vi "LVClass_HasoSlopes ctor from HasoData.vi"(0 "HasoSlopes (new)":refnum<class "HasoSlopes.lvclass">, 5 "HasoData":refnum<class "HasoData.lvclass">, 7 "Slopes?":enum16{"raw_slopes", "processed_slopes"}(ring), 11 "error in (no error)":errorcluster) -> (4 "HasoSlopes (new)":refnum<class "HasoSlopes.lvclass">, 6 "HasoData (dup)":refnum<class "HasoData.lvclass">, 15 "error out":errorcluster)   [LabVIEW 2020, in "HasoSlopes.lvclass"]
uses:
  HasoSlopes.lvclass
  HasoData.lvclass
  Handle creation.ctl
  HasoSlopes.lvclass/HasoSlopes.ctl
  LVClass_HasoData Read HasoData - property.vi
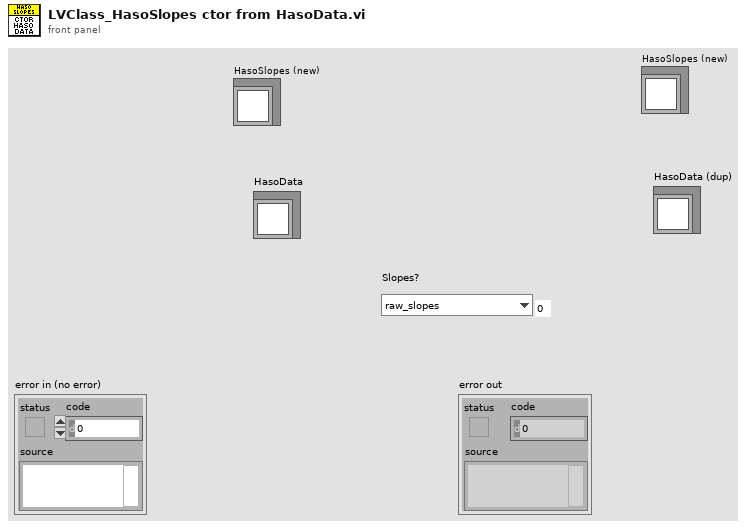
[diagram p1: front panel]
types:
  T1 = typedef "Handle creation.ctl" = enum16{"By ctor", "By write function"}
  T2 = typedef "ClassID.ctl" = i64
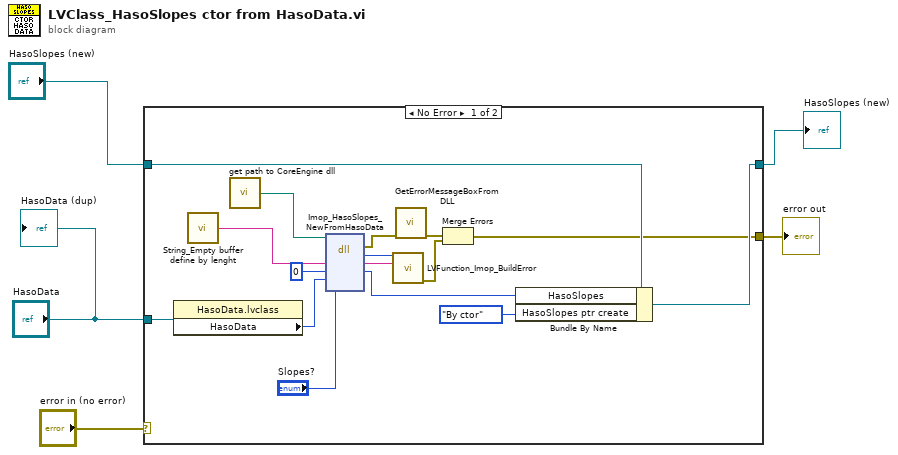
[diagram p0: block diagram]
diagram:
  n1 = case shown="No Error" "error in (no error)" {
    selector: "error in (no error)" -> [_ w23]
    tunnel: [w7 w23] -> w4
    tunnel: [w15 w22] -> w2
    tunnel: "HasoSlopes (new)" -> [w16 w22]
    tunnel: "HasoData" -> [w11 _]
    frame No Error {
      n2 = property class="HasoData.lvclass"(reference=w11) -> ("HasoData"=w10:T2)  [unwired: 1 in, 2 out]
      n3 = call "String_Empty buffer define by lenght.vi"() -> ("Empty buffer"=w17:string)  [unwired: 1 in]
      n4 = call "get path to CoreEngine dll.vi"() -> ("path to wavekit library"=w14:path)  [unwired: 14 in, 1 out]
      n5 = dll-call lib="D:/FLE/0.Code/CoreEngine4_Suite/LV2011_interface/DLLs/c_interface_vc100.dll" fn="Imop_HasoSlopes_NewFromHasoData"(path in=w14, "message"=w17, "objet"=0, "haso data"=w10, "apply_slopes"="Slopes?") -> (error out=w13:errorcluster, "return type"=w20:i32, "message"=w19:string, "objet"=w18:i64)  [unwired: 4 in, 1 out]
      n6 = call "LVFunction_Imop_BuildError.vi"("code"=w20, "String to Prepend to source (\"\")"=w19) -> ("error out"=w8:errorcluster)  [unwired: 13 in]
      n7 = call "GetErrorMessageBoxFromDLL.vi"("error IN"=w13) -> ("error OUT"=w9:errorcluster)  [unwired: 10 in]
      n8 = Merge Errors(w9, w8) -> (w7:errorcluster)
      n9 = Bundle By Name(cluster=w16, "HasoSlopes"=w18, "HasoSlopes ptr create"=Handle_creation."By ctor" ("HasoData ptr create")) -> (w15:refnum<class "HasoSlopes.lvclass">)
    }
    frame Error {
    }
  }
  "error out" <- w4
  "HasoSlopes (new)" <- w2
  "HasoData (dup)" <- "HasoData"
